vi "Mapping Error Dialog.vi"(8 "error in (no error)":errorcluster, 10 "Single Connect?":bool, 11 "Mapping Errors":string[][](array[string])) -> (0 "error out":errorcluster, 3 "Continue?":bool)   [LabVIEW 2016, in "System Mapping Tool.lvlib"]
uses:
  System Mapping Tool.lvlib
  <vilib>/Utility/miscctls.llb/LVRowAndColumnTypeDef.ctl
panel:
  in  "Continue":bool
  in  "Cancel":bool
  in  "Mapping Errors":i32(listbox)
  # "The following mappings are invalid because either the source or destination channels are not valid or because existing mappings conflict with the requsted mappings:"
  # "Would you like to continue importing the remaining mappings?"
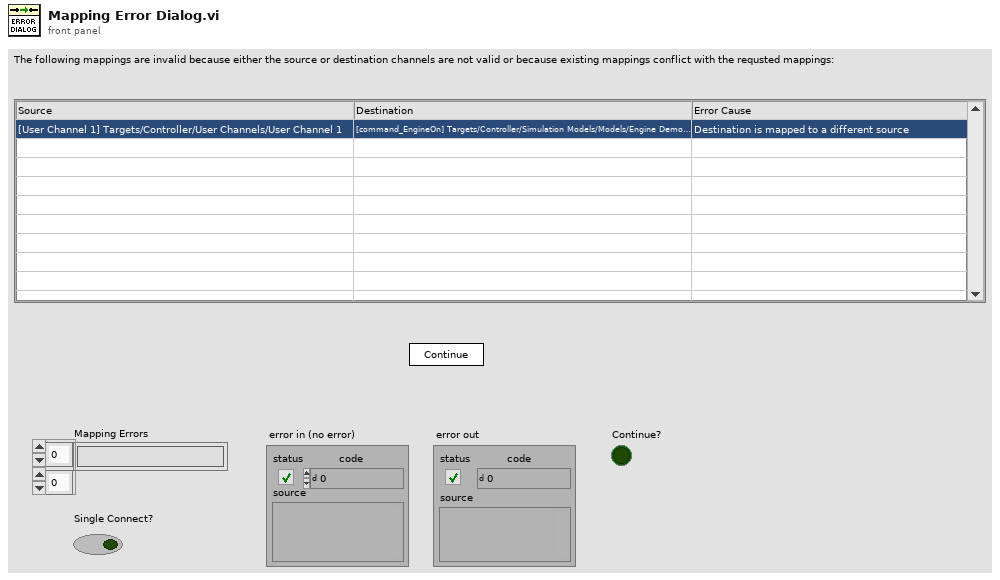
[diagram p1: front panel]
types:
  T1 = typedef "LVRowAndColumnTypeDef.ctl" = cluster{"Row":i32, "Column":i32}
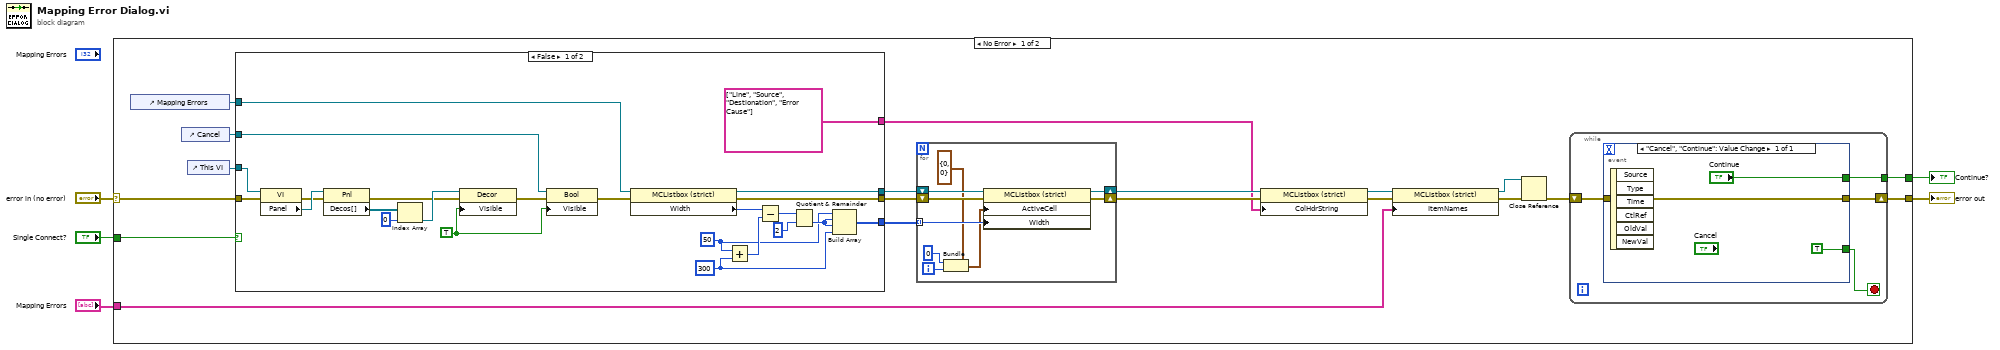
[diagram p0: block diagram]
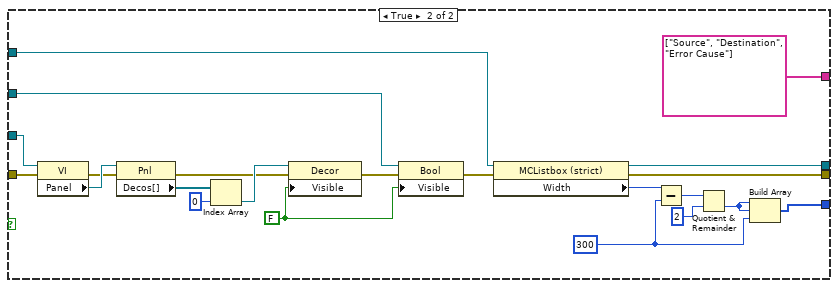
[diagram p2: hidden frame]
diagram:
  n1 = case shown="No Error" "error in (no error)" {
    selector: "error in (no error)" -> [w16 w87]
    tunnel: "Mapping Errors" -> [w22 _]
    tunnel: [w18 w87] -> w3
    tunnel: [w17 _] -> w1
    tunnel: "Single Connect?" -> [w15 _]
    frame No Error {
      n2 = control-ref of="Mapping Errors"() -> (w14:refnum<vi>)
      n3 = control-ref of="Cancel"() -> (w6:refnum<vi>)
      n4 = control-ref of="This VI"() -> (w7:refnum<vi>)
      n5 = case shown="False" w15 {
        tunnel: w16 -> [w48 w68]
        tunnel: w14 -> [w64 w81]
        tunnel: [w56 w78] -> w11
        tunnel: [w55 w80] -> w13
        tunnel: [w54 w79] -> w12
        tunnel: [string[] ["Line", "Source", "Destionation", "Error Cause"] ("Column Header Strings[]") string[] ["Source", "Destination", "Error Cause"] ("Column Header Strings[]")] -> w8
        tunnel: w7 -> [w45 w66]
        tunnel: w6 -> [w44 w65]
        frame False {
          w41 = TRUE ("Visible")
          w58 = u32 300 ("Bounds:Area Width")
          w57 = u32 50 ("Bounds:Area Width")
          n6 = property class="VI"(reference=w45, error in=w48) -> (error out=w47:errorcluster, "Panel"=w49:refnum<vi>)  [unwired: 1 out]
          n7 = property class="Pnl"(reference=w49, error in=w47) -> (error out=w46:errorcluster, "Decos[]"=w50:refnum<vi>[])  [unwired: 1 out]
          n8 = Index Array(array=w50, index=0) -> (element=w51:refnum<vi>)
          n9 = property class="Decor"(reference=w51, error in=w46, "Visible"=w41) -> (error out=w43:errorcluster)  [unwired: 1 out]
          n10 = property class="Bool"(reference=w44, error in=w43, "Visible"=w41) -> (error out=w42:errorcluster)  [unwired: 1 out]
          n11 = property class="MCListbox (strict)"(reference=w64, error in=w42) -> (reference out=w55:refnum<vi>, error out=w54:errorcluster, "Width"=w63:u32)
          n12 = Add(x=w57, y=w58) -> (x+y=w62:u32)
          n13 = Subtract(x=w63, y=w62) -> (x-y=w61:u32)
          n14 = Quotient & Remainder(x=w61, y=u32 2) -> (floor(x/y)=w59:u32)  [unwired: 1 out]
          n15 = Build Array(w57, w59, w59, w58) -> (w56:u32[])
        }
        frame True {
          w69 = FALSE ("Visible")
          w86 = u32 300 ("Bounds:Area Width")
          n16 = property class="VI"(reference=w66, error in=w68) -> (error out=w72:errorcluster, "Panel"=w73:refnum<vi>)  [unwired: 1 out]
          n17 = property class="Pnl"(reference=w73, error in=w72) -> (error out=w71:errorcluster, "Decos[]"=w74:refnum<vi>[])  [unwired: 1 out]
          n18 = Index Array(array=w74, index=0) -> (element=w75:refnum<vi>)
          n19 = property class="Decor"(reference=w75, error in=w71, "Visible"=w69) -> (error out=w70:errorcluster)  [unwired: 1 out]
          n20 = property class="Bool"(reference=w65, error in=w70, "Visible"=w69) -> (error out=w67:errorcluster)  [unwired: 1 out]
          n21 = property class="MCListbox (strict)"(reference=w81, error in=w67) -> (reference out=w80:refnum<vi>, error out=w79:errorcluster, "Width"=w82:u32)
          n22 = Subtract(x=w82, y=w86) -> (x-y=w83:u32)
          n23 = Quotient & Remainder(x=w83, y=u32 2) -> (floor(x/y)=w85:u32)  [unwired: 1 out]
          n24 = Build Array(w85, w85, w86) -> (w78:u32[])
        }
      }
      n25 = for {
        shift-right: [w38] -> w9
        shift-left: w13 -> [w40]
        shift-right: [w37] -> w10
        shift-left: w12 -> [w39]
        tunnel: w11 -> [w36] mode=indexing
        i -> [w35]
        n26 = Bundle(cluster=T1 {"Row"=0, "Column"=0} ("Active Cell:Active Cell"), "Row"=0, "Column"=w35) -> (w33:T1)
        n27 = property class="MCListbox (strict)"(reference=w40, error in=w39, "ActiveCell"=w33, "Width"=w36) -> (reference out=w38:refnum<vi>, error out=w37:errorcluster)
      }
      n28 = property class="MCListbox (strict)"(reference=w9, error in=w10, "ColHdrString"=w8) -> (reference out=w24:refnum<vi>, error out=w23:errorcluster)
      n29 = property class="MCListbox (strict)"(reference=w24, error in=w23, "ItemNames"=w22) -> (reference out=w20:refnum<vi>, error out=w21:errorcluster)
      n30 = Close Reference(reference=w20, error in (no error)=w21) -> (error out=w19:errorcluster)
      n31 = while {
        shift-right: [w27] -> w18
        shift-left: w19 -> [w28]
        tunnel: [w25] -> w17
        stop <- w26 stop-if-true
        n32 = event shown="[0] \"Cancel\", \"Continue\": Value Change" {
          selector: _ -> [_]
          dyn-events: _ -> [_]
          timeout: _ -> [_]
          tunnel: w28 -> [w31]
          tunnel: [w31] -> w27
          tunnel: [TRUE] -> w26
          tunnel: ["Continue"] -> w25
          event "Cancel", "Continue": Value Change {
            n33 = event-data() -> ()  [unwired: 1 in, 6 out]
          }
        }
      }
    }
    frame Error {
    }
  }
  "error out" <- w3
  "Continue?" <- w1
